vi "x1_move4.vi"() -> (0 "Enum":T1(ring))   [LabVIEW 2016]
uses:
  <vilib>/NXT/Block Support/NXT_OutputPort.ctl
  <vilib>/NXT/NXTIO Xnodes/NXTIONodeSubVIs/NXTMotorRunDistance.vi
  <vilib>/NXT/NXTIO Xnodes/NXTIONodeSubVIs/NXTMoveMotors.vi
  <vilib>/NXT/NXTIO Xnodes/NXTIONodeSubVIs/LEGOMotorStatus.vi
  <vilib>/NXT/NXTIO Xnodes/NXTIONodeSubVIs/NXTStopMotors.vi
  <vilib>/NXT/NXTIO Xnodes/NXTIONodeSubVIs/LEGOResetMotors.vi
  <vilib>/NXT/NXTIO Xnodes/AddressXNode/NXTIOAddress.xnode
  <vilib>/NXT/Subs/LVHSConnector.ctl
  <vilib>/NXT/NXTIO Xnodes/NXTIOXNode/NXTIO.xnode
  <vilib>/NXT/LegoClasses/BrickReference/BrickReference.lvclass
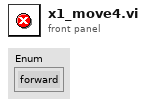
[diagram p1: front panel]
types:
  T1 = enum16{"forward", "right", "mark", "pause", "up", "return", "end"}
  T2 = enum16{"f_r", "up", "u_l", "vorwarts", "ruckwarts", "down", "r_r", "end"}
  T3 = typedef "NXT_OutputPort.ctl" = u8
  T4 = cluster{"Output Port":T3, "Output Port 2":T3, "Output Port 3":T3}
  T5 = typedef "LVHSConnector.ctl" = refnum<class "BrickReference.lvclass">
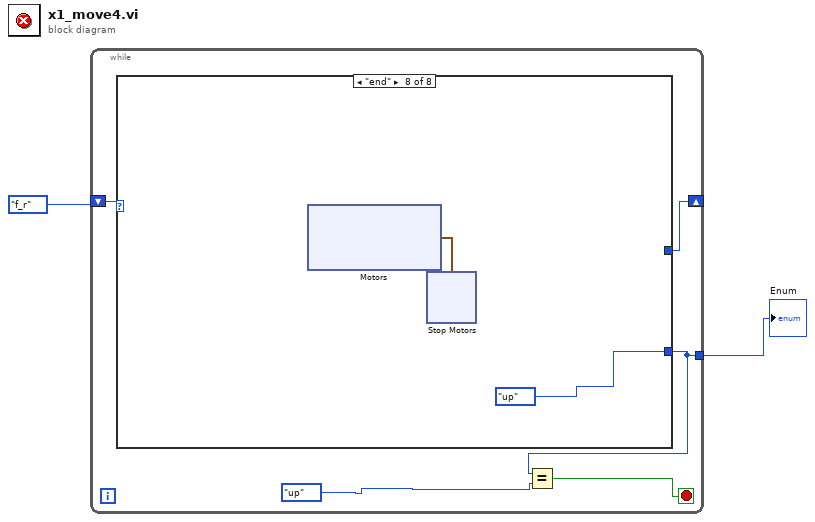
[diagram p0: block diagram]
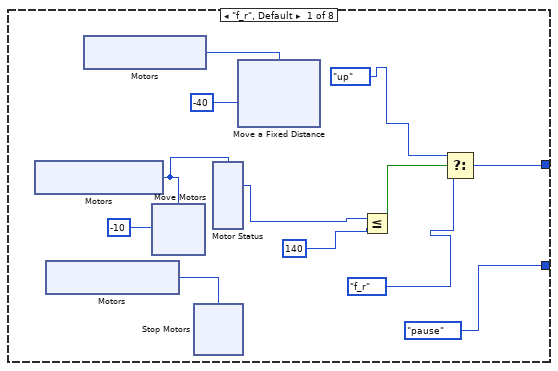
[diagram p2: hidden frame]
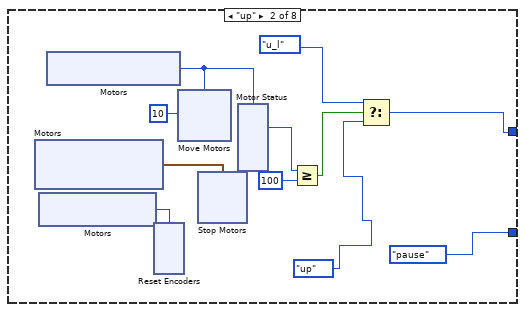
[diagram p3: hidden frame]
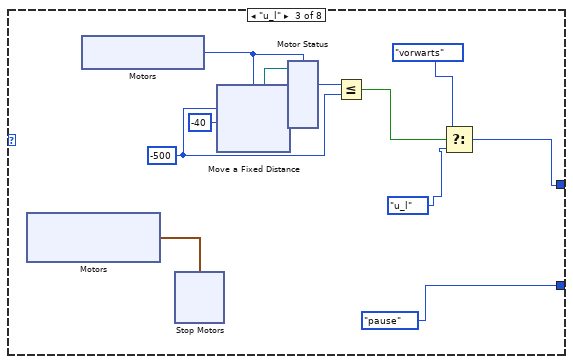
[diagram p4: hidden frame]
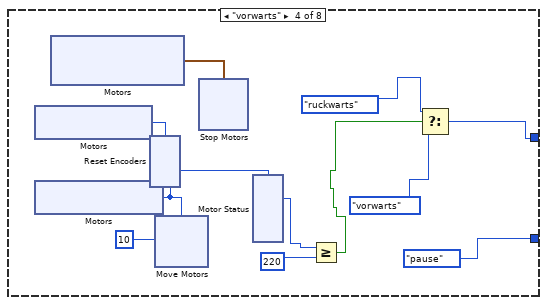
[diagram p5: hidden frame]
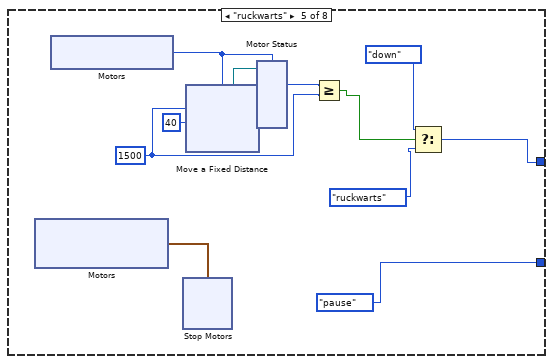
[diagram p6: hidden frame]
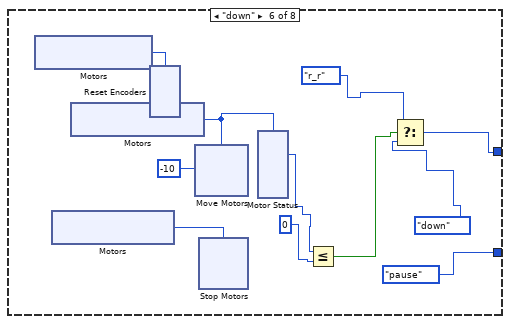
[diagram p7: hidden frame]
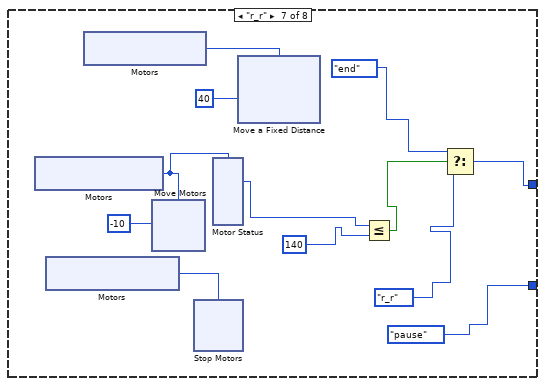
[diagram p8: hidden frame]
diagram:
  n1 = while {
    shift-right: [w4] -> _
    shift-left: T2."f_r" -> [w5]
    tunnel: [w3] -> w1
    stop <- w7 stop-if-true
    n2 = case shown="\"end\"" w5 {
      tunnel: [w14 w56 w91 w134 w165 w204 w245 _] -> w4
      tunnel: [T1."pause" T1."pause" T1."pause" T1."pause" T1."pause" T1."pause" T1."pause" T1."up"] -> w3
      frame "f_r", Default {
        n3 = xnode "Motors"() -> ("Motor"=w16:T3)
        n4 = xnode "Motors"() -> ("Motor"=w15:T3)
        n5 = xnode "Motors"() -> ("Motor"=w18:T3)
        n6 = xnode "Move Motors"("Power/Speed 1"=i8 -10, "Motors"=w16) -> ()  [unwired: 1 in, 1 out]
        n7 = xnode "Stop Motors"("Motors"=w15) -> ()  [unwired: 1 in, 1 out]
        n8 = xnode "Motor Status"("Motors"=w16) -> ("Position 1"=w13:i32)  [unwired: 1 in, 2 out]
        n9 = xnode "Move a Fixed Distance"("Speed 1"=i8 -40, "Motors"=w18) -> ()  [unwired: 2 in, 1 out]
        n10 = Less Or Equal?(x=w13, y=140) -> (x <= y?=w11:bool)
        n11 = Select(t=T2."up", s=w11, f=T2."f_r") -> (s? t:f=w14:T2)
      }
      frame "up" {
        n12 = xnode "Motors"() -> ("Motor"=w62:cluster{"Port":T3, "Port":T3})
        n13 = xnode "Motors"() -> ("Motor"=w57:T3)
        n14 = xnode "Motors"() -> ("Motor"=w59:T3)
        n15 = xnode "Reset Encoders"("Motors"=w57) -> ()  [unwired: 1 in, 1 out]
        n16 = xnode "Move Motors"("Power/Speed 1"=i8 10, "Motors"=w59) -> ()  [unwired: 1 in, 1 out]
        n17 = xnode "Stop Motors"("Motors"=w62) -> ()  [unwired: 1 in, 1 out]
        n18 = xnode "Motor Status"("Motors"=w59) -> ("Position 1"=w60:i32)  [unwired: 1 in, 2 out]
        n19 = Greater Or Equal?(x=w60, y=100) -> (x >= y?=w61:bool)
        n20 = Select(t=T2."u_l", s=w61, f=T2."up") -> (s? t:f=w56:T2)
      }
      frame "u_l" {
        w98 = -500 ("Distance 1")
        n21 = xnode "Motors"() -> ("Motor"=w101:cluster{"Port":T3, "Port":T3})
        n22 = xnode "Motors"() -> ("Motor"=w96:T3)
        n23 = xnode "Stop Motors"("Motors"=w101) -> ()  [unwired: 1 in, 1 out]
        n24 = xnode "Move a Fixed Distance"("Speed 1"=i8 -40, "Distance 1"=w98, "Motors"=w96) -> ("NXT/EV3"=w95:T5)  [unwired: 1 in]
        n25 = xnode "Motor Status"("Motors"=w96, "NXT/EV3"=w95) -> ("Position 1"=w99:i32)  [unwired: 2 out]
        n26 = Less Or Equal?(x=w99, y=w98) -> (x <= y?=w97:bool)
        n27 = Select(t=T2."vorwarts", s=w97, f=T2."u_l") -> (s? t:f=w91:T2)
      }
      frame "vorwarts" {
        n28 = xnode "Motors"() -> ("Motor"=w129:T3)
        n29 = xnode "Motors"() -> ("Motor"=w136:T3)
        n30 = xnode "Motors"() -> ("Motor"=w135:cluster{"Port":T3, "Port":T3})
        n31 = xnode "Reset Encoders"("Motors"=w129) -> ()  [unwired: 1 in, 1 out]
        n32 = xnode "Move Motors"("Power/Speed 1"=i8 10, "Motors"=w136) -> ()  [unwired: 1 in, 1 out]
        n33 = xnode "Stop Motors"("Motors"=w135) -> ()  [unwired: 1 in, 1 out]
        n34 = xnode "Motor Status"("Motors"=w136) -> ("Position 1"=w133:i32)  [unwired: 1 in, 2 out]
        n35 = Greater Or Equal?(x=w133, y=220) -> (x >= y?=w131:bool)
        n36 = Select(t=T2."ruckwarts", s=w131, f=T2."vorwarts") -> (s? t:f=w134:T2)
      }
      frame "ruckwarts" {
        w169 = 1500 ("Distance 1")
        n37 = xnode "Motors"() -> ("Motor"=w174:cluster{"Port":T3, "Port":T3})
        n38 = xnode "Motors"() -> ("Motor"=w172:T3)
        n39 = xnode "Stop Motors"("Motors"=w174) -> ()  [unwired: 1 in, 1 out]
        n40 = xnode "Move a Fixed Distance"("Speed 1"=i8 40, "Distance 1"=w169, "Motors"=w172) -> ("NXT/EV3"=w171:T5)  [unwired: 1 in]
        n41 = xnode "Motor Status"("Motors"=w172, "NXT/EV3"=w171) -> ("Position 1"=w170:i32)  [unwired: 2 out]
        n42 = Greater Or Equal?(x=w170, y=w169) -> (x >= y?=w168:bool)
        n43 = Select(t=T2."down", s=w168, f=T2."ruckwarts") -> (s? t:f=w165:T2)
      }
      frame "down" {
        n44 = xnode "Motors"() -> ("Motor"=w207:T3)
        n45 = xnode "Motors"() -> ("Motor"=w211:T3)
        n46 = xnode "Motors"() -> ("Motor"=w209:T3)
        n47 = xnode "Reset Encoders"("Motors"=w207) -> ()  [unwired: 1 in, 1 out]
        n48 = xnode "Move Motors"("Power/Speed 1"=i8 -10, "Motors"=w209) -> ()  [unwired: 1 in, 1 out]
        n49 = xnode "Stop Motors"("Motors"=w211) -> ()  [unwired: 1 in, 1 out]
        n50 = xnode "Motor Status"("Motors"=w209) -> ("Position 1"=w208:i32)  [unwired: 1 in, 2 out]
        n51 = Less Or Equal?(x=w208, y=0) -> (x <= y?=w205:bool)
        n52 = Select(t=T2."r_r", s=w205, f=T2."down") -> (s? t:f=w204:T2)
      }
      frame "r_r" {
        n53 = xnode "Motors"() -> ("Motor"=w247:T3)
        n54 = xnode "Motors"() -> ("Motor"=w246:T3)
        n55 = xnode "Motors"() -> ("Motor"=w249:T3)
        n56 = xnode "Move Motors"("Power/Speed 1"=i8 -10, "Motors"=w247) -> ()  [unwired: 1 in, 1 out]
        n57 = xnode "Stop Motors"("Motors"=w246) -> ()  [unwired: 1 in, 1 out]
        n58 = xnode "Motor Status"("Motors"=w247) -> ("Position 1"=w243:i32)  [unwired: 1 in, 2 out]
        n59 = xnode "Move a Fixed Distance"("Speed 1"=i8 40, "Motors"=w249) -> ()  [unwired: 2 in, 1 out]
        n60 = Less Or Equal?(x=w243, y=140) -> (x <= y?=w241:bool)
        n61 = Select(t=T2."end", s=w241, f=T2."r_r") -> (s? t:f=w245:T2)
      }
      frame "end" {
        n62 = xnode "Motors"() -> ("Motor"=w285:cluster{"Port":T3, "Port":T3, "Port":T3})
        n63 = xnode "Stop Motors"("Motors"=w285) -> ()  [unwired: 1 in, 1 out]
      }
    }
    n64 = Equal?(x=w3, y=T1."up") -> (x = y?=w7:bool)
  }
  "Enum" <- w1
